vi "Time String Formatter.vi"(1 "Time":timestamp format="%<%x %.3X>T") -> (0 "Time string":string)   [LabVIEW 2019, in "TSC Event Logger.lvlib" / "Layout.lvclass"]
doc: "Format time string into ISO-8601\n\nhttps://en.wikipedia.org/wiki/ISO_8601\n\n<b>Code Developed By:</b>\nTechnology Service Corporation\nBloomington, IN 47403\nwww.tsc.com/atcs\n\nDeveloper:\nDaniel Coons"
uses:
  Layout.lvclass
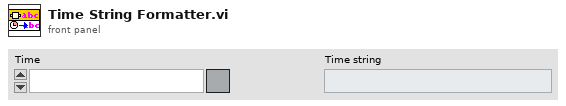
[diagram p1: front panel]
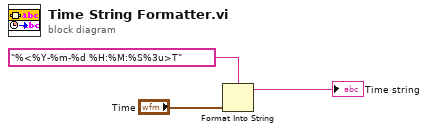
[diagram p0: block diagram]
diagram:
  n1 = Format Into String(format string="%<%Y-%m-%d %H:%M:%S%3u>T", "Time") -> (resulting string=→"Time string":string)  [unwired: 2 in, 1 out]
